vi "test Largest Channel Array.vi"(8 "error in (no error)":errorcluster, 11 "TestCase in":refnum<class "Configuration Tests.lvclass">) -> (0 "error out":errorcluster, 3 "TestCase out":refnum<class "Configuration Tests.lvclass">)   [LabVIEW 2017, in "Configuration Tests.lvclass"]
uses:
  Configuration Tests.lvclass
  <vilib>/addons/_JKI Toolkits/VI Tester/TestCase.llb/TestCase.lvclass
  Mock Classes/Transfer/Mock Transfer.lvclass
  Typedefs/DSF Data Type.ctl
  DSF Core.lvlib
  Typedefs/DSF Engine Channel Configuration.ctl
  Mock Classes/Transfer Group/Mock Transfer Group.lvclass
  C:/Git/DSF/Data Sharing Framework Core/Classes/Transfer/Transfer.lvclass
  C:/Program Files (x86)/National Instruments/LabVIEW 2017/vi.lib/addons/_JKI Toolkits/VI Tester/TestCase.llb/TestCase.lvclass
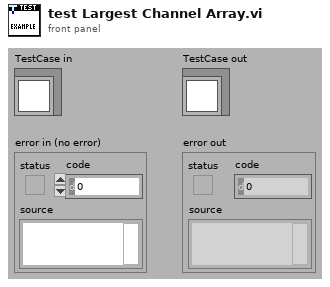
[diagram p1: front panel]
types:
  T1 = typedef "DSF Core.lvlib/DSF Engine Channel Configuration.ctl" = cluster{"engine offset":u64, "name":string, "data type":T2, "count":u64, "buffer offset":u64}
  T2 = typedef "DSF Core.lvlib/DSF Data Type.ctl" = enum8{"Bool", "SGL", "DBL", "I8", "I16", "I32", "I64", "U8", "U16", "U32", "U64"}
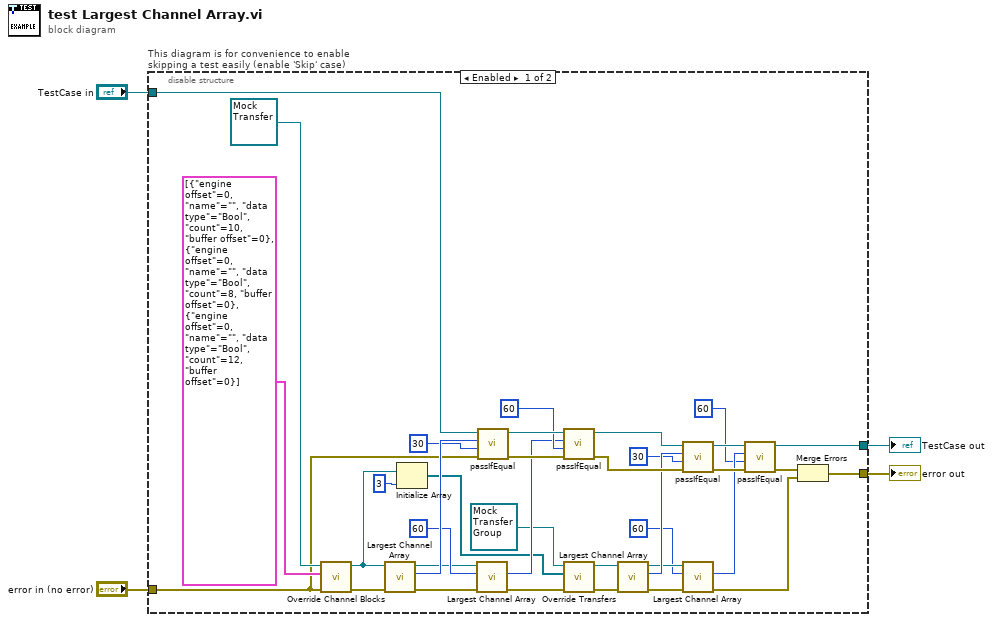
[diagram p0: block diagram]
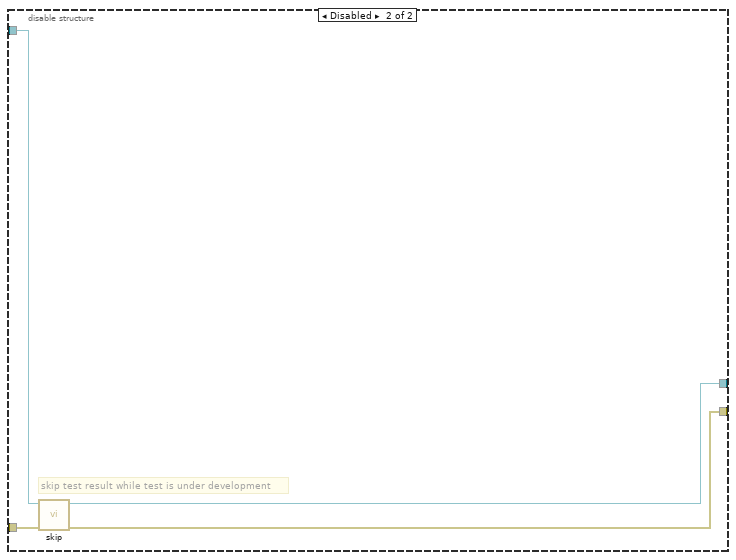
[diagram p2: hidden frame]
diagram:
  n1 = disable-structure "This diagram is for convenience to enable skipping a test easily (enable 'Skip' case)" shown="Enabled" {
    disable-tunnel: "TestCase in" -> [w36 w44]
    disable-tunnel: [w10 w42] -> w1
    disable-tunnel: [w37 w43] -> w3
    disable-tunnel: "error in (no error)" -> [w32 w41]
    frame Enabled {
      n2 = call "Override Channel Blocks.vi"("error in (no error)"=w32, "channel blocks"=T1[] [{"engine offset"=0, "name"="", "data type"=enum."Bool", "count"=10, "buffer offset"=0}, {"engine offset"=0, "name"="", "data type"=enum."Bool", "count"=8, "buffer offset"=0}, {"engine offset"=0, "name"="", "data type"=enum."Bool", "count"=12, "buffer offset"=0}], "Mock Transfer in"=refnum<class "Mock Transfer.lvclass"> refnum ("Mock Transfer.lvclass")) -> ("error out"=w38:errorcluster, "Mock Transfer out"=w24:refnum<class "Mock Transfer.lvclass">)  [unwired: 7 in]
      n3 = call "Largest Channel Array.vi"("error in (no error)"=w38, "Transfer in"=w24) -> ("error out"=w29:errorcluster, "largest channel array out"=w35:u64, "Transfer out"=w5:refnum<class "Mock Transfer.lvclass">)  [unwired: 7 in]
      n4 = Initialize Array(w24, 3 ("dimension size")) -> (w22:refnum<class "Mock Transfer.lvclass">[])
      n5 = call "Largest Channel Array.vi"("error in (no error)"=w29, "largest channel array in (0)"=u64 60, "Transfer in"=w5) -> ("error out"=w16:errorcluster, "largest channel array out"=w26:u64)  [unwired: 6 in, 1 out]
      n6 = call-dynamic "passIfEqual.vi"("error in (no error)"=w32, "y"=u64 30 ("largest channel array out"), "x"=w35, "TestCase in"=w36) -> ("error out"=w33:errorcluster, "TestCase out"=w30:refnum<class "Configuration Tests.lvclass">)  [unwired: 6 in]
      n7 = call-dynamic "passIfEqual.vi"("error in (no error)"=w33, "y"=u64 60 ("largest channel array out"), "x"=w26, "TestCase in"=w30) -> ("error out"=w31:errorcluster, "TestCase out"=w19:refnum<class "Configuration Tests.lvclass">)  [unwired: 6 in]
      n8 = call "Override Transfers.vi"("error in (no error)"=w16, "Transfers"=w22, "Mock Transfer Group in"=refnum<class "Mock Transfer Group.lvclass"> refnum ("Mock Transfer Group.lvclass")) -> ("error out"=w15:errorcluster, "Mock Transfer Group out"=w21:refnum<class "Mock Transfer Group.lvclass">)  [unwired: 7 in]
      n9 = call "Largest Channel Array.vi"("error in (no error)"=w15, "Transfer Group in"=w21) -> ("error out"=w6:errorcluster, "largest channel array out"=w18:u64, "Transfer Group out"=w14:refnum<class "Mock Transfer Group.lvclass">)  [unwired: 7 in]
      n10 = call-dynamic "passIfEqual.vi"("error in (no error)"=w31, "y"=u64 30 ("largest channel array out"), "x"=w18, "TestCase in"=w19) -> ("error out"=w20:errorcluster, "TestCase out"=w11:refnum<class "Configuration Tests.lvclass">)  [unwired: 6 in]
      n11 = call "Largest Channel Array.vi"("error in (no error)"=w6, "largest channel array in (0)"=u64 60, "Transfer Group in"=w14) -> ("error out"=w7:errorcluster, "largest channel array out"=w9:u64)  [unwired: 6 in, 1 out]
      n12 = call-dynamic "passIfEqual.vi"("error in (no error)"=w20, "y"=u64 60 ("largest channel array in (0)"), "x"=w9, "TestCase in"=w11) -> ("error out"=w12:errorcluster, "TestCase out"=w10:refnum<class "Configuration Tests.lvclass">)  [unwired: 6 in]
      n13 = Merge Errors(w12, w7) -> (w37:errorcluster)
    }
    frame Disabled {
      # "skip test result while test is under development"
      n14 = call <vilib>:"skip.vi"("error in (no error)"=w41, "TestCase in"=w44) -> ("error out"=w43:errorcluster, "TestCase out"=w42:refnum<class "Configuration Tests.lvclass">)  [unwired: 8 in]
    }
  }
  "error out" <- w3
  "TestCase out" <- w1
